vi "Lauda_out_09.vi"(11 "params":dbl[](array[numeric])) -> (1 "Elapsed":i32, 2 "Tr":dbl, 4 "Current step":i32, 7 "T control":dbl, 10 "T set":dbl)   [LabVIEW 2015]
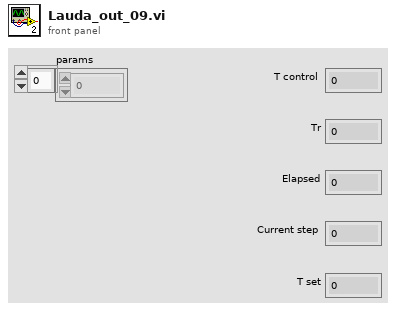
[diagram p1: front panel]
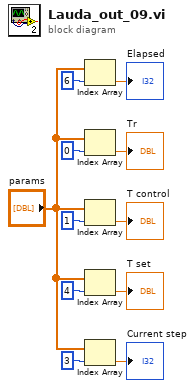
[diagram p0: block diagram]
diagram:
  n1 = Index Array(array="params", index=6) -> (element=→"Elapsed":dbl)
  n2 = Index Array(array="params", index=0) -> (element=→"Tr":dbl)
  n3 = Index Array(array="params", index=1) -> (element=→"T control":dbl)
  n4 = Index Array(array="params", index=4) -> (element=→"T set":dbl)
  n5 = Index Array(array="params", index=3) -> (element=→"Current step":dbl)
